vi "Add Message to Transmit Schedule.vi"() -> ()   [LabVIEW 2019]
doc: "This example program opens the specified device, finds the first available core and first available ARINC 429 transmit channel. It then configures that transmit \nchannel with one scheduled message, and monitors that channel for all labels. All monitored labels are listed along with their latest seen timestamp. The \"Add New Message\" button allows the user to insert a new label into the schedule. Once this happens the new label will be displayed by the monitor display. After the new label is added, the \"Add New Message\" button is disabled preventing duplicate messages from being added to the running schedule."
uses:
  <instrlib>/BTI429Lib/Public/Controls/429 Scheduled Message Type.ctl
  <instrlib>/BTICardLib/Private/Initialize By Card Number and Core Number.vi
  <instrlib>/BTICardLib/Private/Configure Core From XML.vi
  <instrlib>/BTI429Lib/Private/Tx/Configure/Configure Tx Channel From XML.vi
  <instrlib>/BTI429Lib/Private/Core/Action-Status/Start All Channels.vi
  <instrlib>/BTI429Lib/Private/Utility/Get Fld Label.vi
  <instrlib>/BTI429Lib/Private/Core/Action-Status/Stop All Channels.vi
  <instrlib>/BTI429Lib/BTI429LV.lvlib
  <instrlib>/BTICardLib/BTICardLV.lvlib
panel:
  out "Labels":u16[](array[numeric]) format="%o"
  out "Timestamps":u32[](array[numeric]) format="%x"
  in  "Add New Message":bool
  out "core number":i32
  out "channel number":i32
  out "error out":errorcluster
  in  "stop":bool
  in  "Channel XML Configuration":string="Channel Config.xml"
  in  "Core XML Configuration":string="Core Config.xml"
  in  "Card Number":i32
  # "ARINC 429: Add Message to Transmit Schedule"
  # "©2016 Astronics Ballard Technology"
  # "This example program opens the specified device, finds the first available core and first available ARINC 429 transmit channel. It then configures that transmit \nchannel with one scheduled message, and monitors that channel for all labels. All monitored labels are listed along with their latest seen timestamp. The \"Add New Message\" button allows the user to insert a new label into the schedule. Once this happens the new label will be displayed by the monitor display. After the new label is added, the \"Add New Message\" button is disabled preventing duplicate messages from being added to the running schedule."
  # "Clicking on the \"Add New Message\" button will insert a new label into the running schedule. Once this is done, the button is disbalbled until the Stop button is pressed."
  # "Always Stop the card\nand Close the card when\ndone. Otherwise, the hardware\ncontinues to operate."
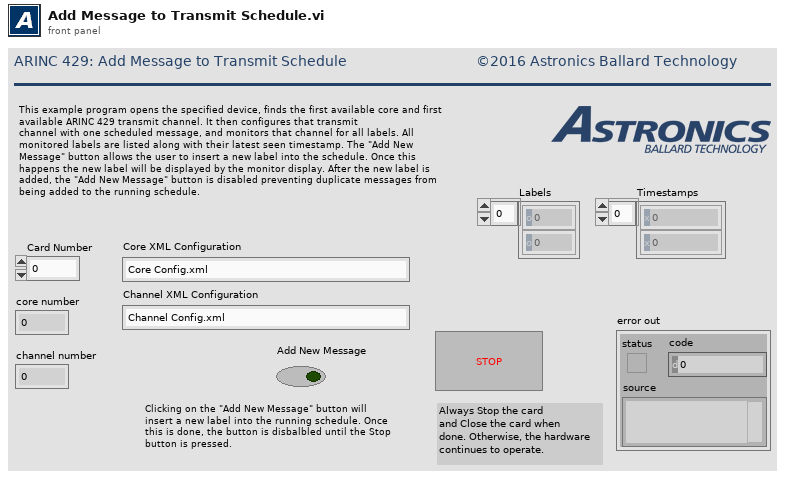
[diagram p1: front panel]
types:
  T1 = enum8{"Enabled", "Disabled", "Disabled and Grayed Out"}
  T2 = typedef "BTI429LV.lvlib/429 Scheduled Message Type.ctl" = u32
  T3 = typedef "BTI429LV.lvlib/429 Record.ctl" = cluster{"type":u16, "count":u16, "timestamp":u32, "msgact":u16, "decgap":u16, "data":u32, "timestamph":u32}
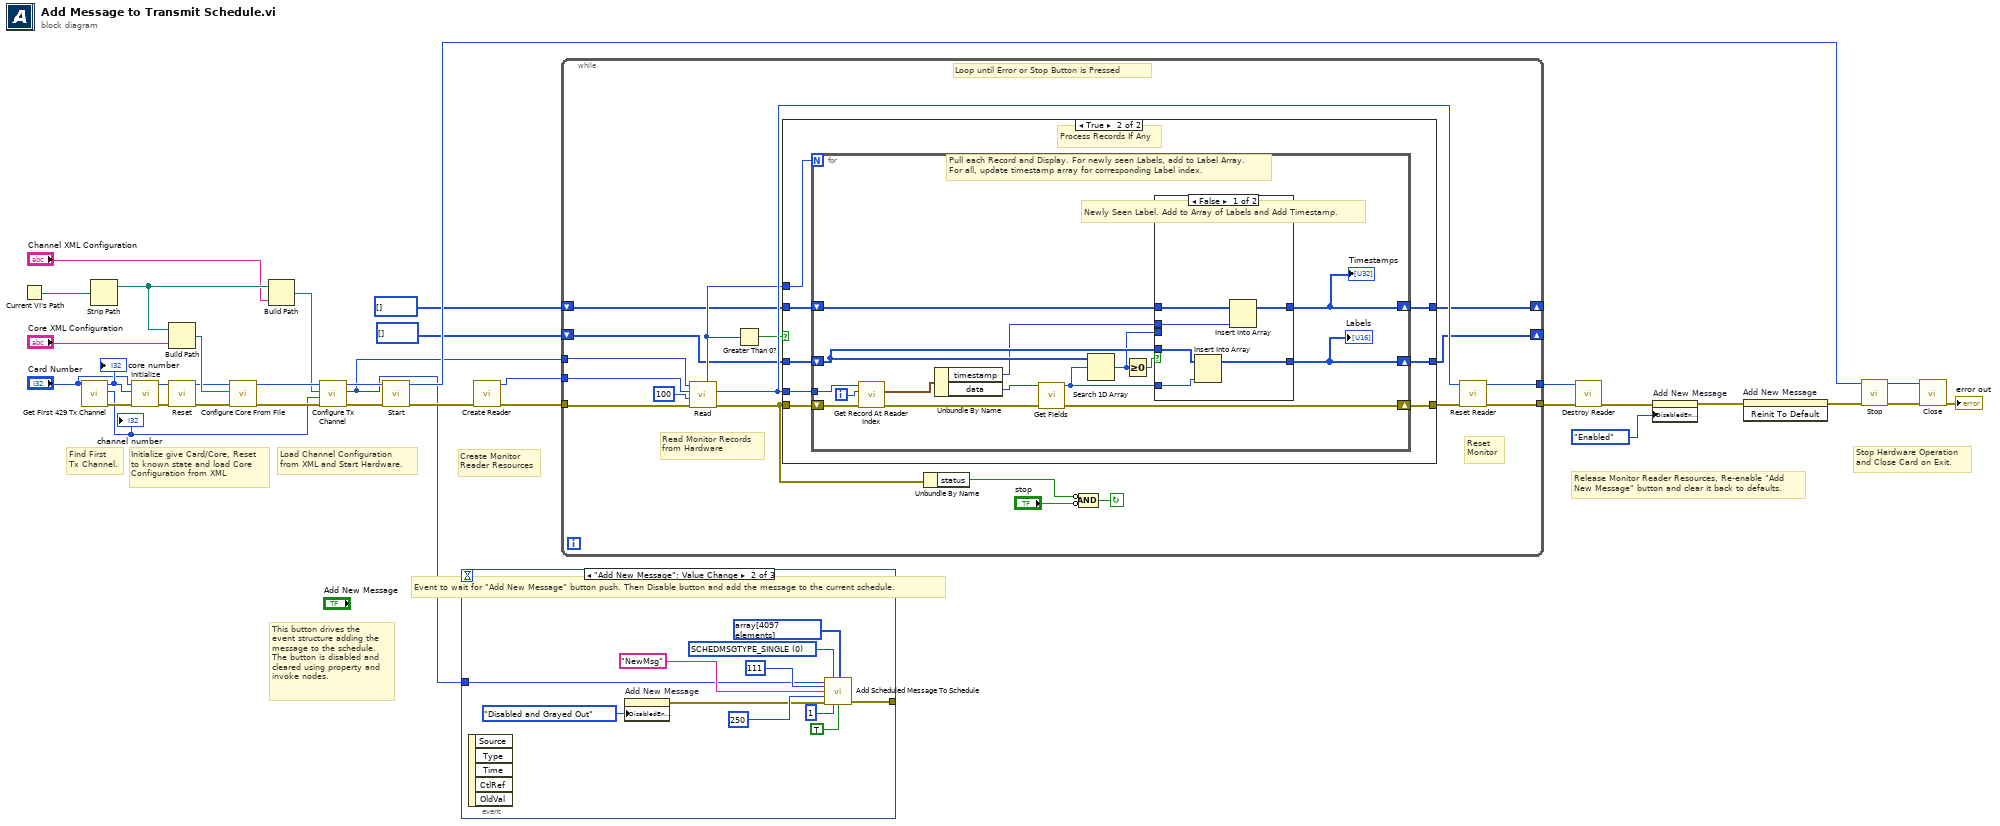
[diagram p0: block diagram]
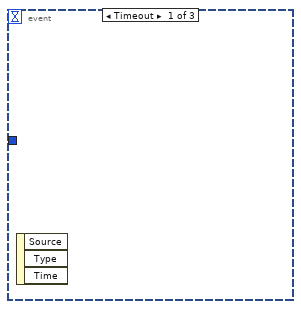
[diagram p2: hidden frame]
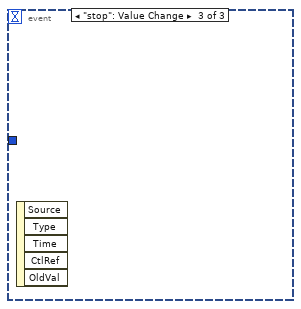
[diagram p3: hidden frame]
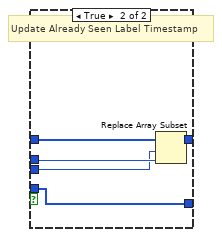
[diagram p5: hidden frame]
diagram:
  # "Release Monitor Reader Resources, Re-enable \"Add\nNew Message\" button and clear it back to defaults."
  # "Create Monitor\nReader Resources"
  # "This button drives the\nevent structure adding the\nmessage to the schedule.\nThe button is disabled and\ncleared using property and\ninvoke nodes."
  # "Find First\nTx Channel."
  # "Load Channel Configuration\nfrom XML and Start Hardware."
  # "Initialize give Card/Core, Reset\nto known state and load Core\nConfiguration from XML"
  # "Stop Hardware Operation\nand Close Card on Exit."
  n1 = Current VI's Path() -> (path=w29:path)
  n2 = call "Get First 429 Tx Channel.vi"("Card Number"="Card Number") -> ("error out"=w14:errorcluster, "Channel Number"=w13:i32, "Core Number"=w16:i32)  [unwired: 8 in]
  "channel number" <- w13
  "core number" <- w16
  n3 = Strip Path(path=w29) -> (stripped path=w28:path)  [unwired: 1 out]
  n4 = call-poly <instrlib>:"Initialize.vi"("error in (no error)"=w14, "core number"=w16, "card number"="Card Number") -> ("error out"=w18:errorcluster, "core handle out"=w19:u64)  [unwired: 7 in]
  n5 = Build Path(base path=w28, name or relative path="Core XML Configuration") -> (appended path=w26:path)
  n6 = call <instrlib>:"Reset.vi"("error in (no error)"=w18, "core handle in"=w19) -> ("error out"=w17:errorcluster, "core handle out"=w20:u64)  [unwired: 8 in]
  n7 = call-poly <instrlib>:"Configure Core From File.vi"("error in (no error)"=w17, "configuration file path"=w26, "core handle in"=w20) -> ("error out"=w33:errorcluster, "core handle out"=w34:u64)  [unwired: 7 in]
  n8 = Build Path(base path=w28, name or relative path="Channel XML Configuration") -> (appended path=w24:path)
  n9 = call-poly <instrlib>:"Configure Tx Channel.vi"("error in (no error)"=w33, "channel number in"=w13, "configuration file path"=w24, "core handle in"=w34) -> ("error out"=w32:errorcluster, "channel handle out"=w5:u64, "core handle out"=w31:u64)  [unwired: 5 in]
  n10 = call-poly <instrlib>:"Start.vi"("error in (no error)"=w32, "core handle in"=w31) -> ("error out"=w9:errorcluster, "core handle out"=w21:u64)  [unwired: 8 in]
  n11 = event shown="[1] \"Add New Message\": Value Change" {
    selector: _ -> [_ _ _]
    dyn-events: _ -> [_ _ _]
    timeout: _ -> [_ _ _]
    tunnel: w5 -> [_ w38 _]
    tunnel: [_ w35 _] -> _
    event Timeout {
      n12 = event-data() -> ()  [unwired: 1 in, 3 out]
    }
    event "Add New Message": Value Change {
      w45 = T2 0 items=["SCHEDMSGTYPE_SINGLE", "SCHEDMSGTYPE_LISTFIFO", "SCHEDMSGTYPE_LISTCIRCULAR"] ("message type")
      # "Event to wait for \"Add New Message\" button push. Then Disable button and add the message to the current schedule."
      n13 = event-data() -> ()  [unwired: 1 in, 5 out]
      n14 = property on="Add New Message" class="Bool"("DisabledEnum"=T1."Disabled and Grayed Out" ("Disabled")) -> (error out=w37:errorcluster)  [unwired: 2 in, 1 out]
      n15 = call <instrlib>:"Add Scheduled Message To Schedule.vi"("channel handle in"=w38, "message type"=w45, "message data"=u32[] array[4097 elements], "message id"=111, "message name"="NewMsg", "message period"=250, "error in (no error)"=w37, "message data count"=1, "monitor message?"=TRUE) -> ("error out"=w35:errorcluster)  [unwired: 4 in, 2 out]
    }
    event "stop": Value Change {
      n16 = event-data() -> ()  [unwired: 1 in, 5 out]
    }
  }
  n17 = call <instrlib>:"Create Reader.vi"("error in (no error)"=w9) -> ("error out"=w10:errorcluster, "reader handle out"=w8:u64)  [unwired: 9 in]
  n18 = while {
    tunnel: w5 -> [w48]
    tunnel: w10 -> [w55]
    tunnel: [w54] -> w7
    tunnel: [w53] -> w6
    shift-right: [w50] -> _
    shift-left: u32[] [] -> [w52]
    shift-right: [w49] -> _
    shift-left: u16[] [] -> [w51]
    tunnel: w8 -> [w47]
    stop <- w63 continue-if-true
    # "Reset\nMonitor"
    # "Read Monitor Records\nfrom Hardware"
    # "Loop until Error or Stop Button is Pressed"
    n19 = call <instrlib>:"Read.vi"("error in (no error)"=w55, "max records to read"=100, "reader handle in"=w47, "channel handle in"=w48) -> ("error out"=w46:errorcluster, "reader handle out"=w59:u64, "records read"=w58:i32)  [unwired: 3 in, 2 out]
    n20 = Greater Than 0?(x=w58) -> (x > 0?=w57:bool)
    n21 = case shown="True" w57 {
      tunnel: w59 -> [_ w74]
      tunnel: w58 -> [_ w73]
      tunnel: w46 -> [w66 w71]
      tunnel: [w66 w72] -> w60
      tunnel: w51 -> [w64 w70]
      tunnel: w52 -> [w65 w68]
      tunnel: [w65 w69] -> w50
      tunnel: [w64 w67] -> w49
      frame False {
      }
      frame True {
        # "Process Records If Any"
        n22 = for {
          N: w73 -> [_]
          tunnel: w74 -> [w89]
          shift-right: [w84] -> w72
          shift-left: w71 -> [w87]
          shift-right: [w80] -> w67
          shift-left: w70 -> [w79]
          shift-right: [w77] -> w69
          shift-left: w68 -> [w76]
          i -> [w88]
          # "Pull each Record and Display. For newly seen Labels, add to Label Array.\nFor all, update timestamp array for corresponding Label index."
          n23 = call <instrlib>:"Get Record At Reader Index.vi"("error in (no error)"=w87, "record index"=w88, "reader handle in"=w89) -> ("error out"=w85:errorcluster, "record out"=w86:T3)  [unwired: 6 in, 1 out]
          n24 = Unbundle By Name(w86) -> ("timestamp"=w78:u32, "data"=w83:u32)
          n25 = call-poly <instrlib>:"Get Fields.vi"("error in (no error)"=w85, "message"=w83) -> ("error out"=w84:errorcluster, "label out"=w81:u16)  [unwired: 8 in]
          n26 = Search 1D Array(1D array=w79, element=w81) -> (index of element=w75:i32)  [unwired: 1 in]
          n27 = Greater Or Equal To 0?(x=w75) -> (x >= 0?=w82:bool)
          n28 = case shown="False" w82 {
            tunnel: w81 -> [w95 _]
            tunnel: w79 -> [w94 w100]
            tunnel: [w93 w100] -> w80
            tunnel: w78 -> [w92 w97]
            tunnel: w76 -> [w91 w98]
            tunnel: [w90 w99] -> w77
            tunnel: w75 -> [_ w96]
            frame False {
              # "Newly Seen Label. Add to Array of Labels and Add Timestamp."
              n29 = Insert Into Array(array=w94, new element=w95) -> (w93:u16[])  [unwired: 1 in]
              n30 = Insert Into Array(array=w91, new element=w92) -> (w90:u32[])  [unwired: 1 in]
            }
            frame True {
              # "Update Already Seen Label Timestamp"
              n31 = Replace Array Subset(array=w98, new element=w97, index=w96) -> (w99:u32[])
            }
          }
          "Timestamps" <- w77
          "Labels" <- w80
        }
      }
    }
    n32 = Unbundle By Name(w46) -> ("status"=w61:bool)
    n33 = Compound Arithmetic op=AND(invert w61, invert "stop") -> (w63:bool)
    n34 = call <instrlib>:"Reset Reader.vi"("error in (no error)"=w60, "reader handle in"=w59) -> ("error out"=w54:errorcluster, "reader handle out"=w53:u64)  [unwired: 8 in]
  }
  n35 = call <instrlib>:"Destroy Reader.vi"("error in (no error)"=w7, "reader handle in"=w6) -> ("error out"=w3:errorcluster)  [unwired: 8 in, 1 out]
  n36 = property on="Add New Message" class="Bool"(error in=w3, "DisabledEnum"=T1."Enabled" ("Disabled")) -> (error out=w2:errorcluster)  [unwired: 1 in, 1 out]
  n37 = invoke on="Add New Message" class="Bool" method="Reinit To Default"(error in=w2) -> (error out=w1:errorcluster)  [unwired: 2 in, 2 out]
  n38 = call-poly <instrlib>:"Stop.vi"("error in (no error)"=w1, "core handle in"=w21) -> ("error out"=w23:errorcluster, "core handle out"=w22:u64)  [unwired: 8 in]
  n39 = call <instrlib>:"Close.vi"("error in (no error)"=w23, "core handle in"=w22) -> ("error out"=→"error out":errorcluster)  [unwired: 8 in, 1 out]
